vi "Update.vi"(8 "error in (no error)":errorcluster, 11 "Example Source in":refnum<class "Example Source.lvclass">) -> (0 "error out":errorcluster, 3 "Example Source out":refnum<class "Example Source.lvclass">)   [LabVIEW 2020, in "Example Source.lvlib" / "Example Source.lvclass"]
uses:
  Example Source.lvclass
  C:/Program Files/National Instruments/LabVIEW 2020/vi.lib/ActorFramework/Actor/Actor.lvclass
  Timestamp/Timestamp.lvclass
  C:/Users/huipeng8/Desktop/Event-Source-Actor/Source/Template Source/Event Data/Event Data.lvclass
  Doublo Array/Doublo Array.lvclass
  <vilib>/ActorFramework/Actor/Actor.lvclass/Actor.ctl
  <vilib>/ActorFramework/Message Enqueuer/Message Enqueuer.lvclass/Message Enqueuer.ctl
  Timestamp/Timestamp.lvclass/Timestamp.ctl
  Doublo Array/Doublo Array.lvclass/Doublo Array.ctl
  Source/Template Source/Event Source Messages/Generate Event Msg/Generate Event Msg.lvclass/Generate Event Msg.ctl
  <vilib>/ActorFramework/Message Enqueuer/Init from Existing Queue.vi
  <vilib>/ActorFramework/Message Enqueuer/Enqueue.vi
  Source/Template Source/Event Source Messages/Generate Event Msg/Generate Event Msg.lvclass
  C:/Program Files/National Instruments/LabVIEW 2020/vi.lib/ActorFramework/Message/Message.lvclass
  <vilib>/ActorFramework/Message Priority Queue/Priority Enqueue.vi
  <vilib>/ActorFramework/Message Enqueuer/Message Enqueuer.lvclass
  <vilib>/ActorFramework/Actor/Actor.lvclass
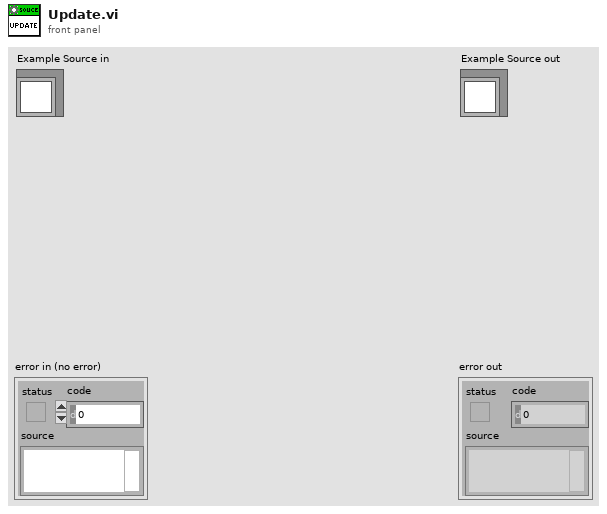
[diagram p1: front panel]
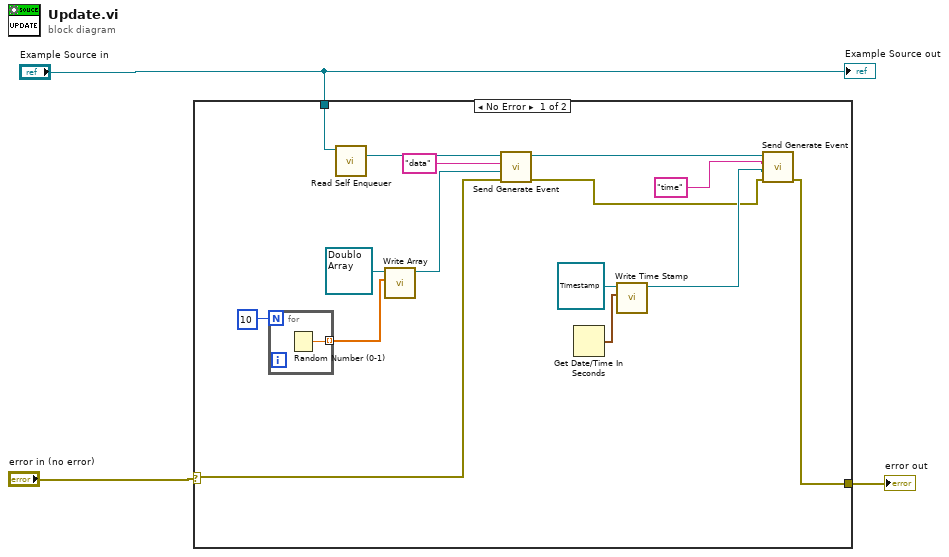
[diagram p0: block diagram]
diagram:
  n1 = case shown="No Error" "error in (no error)" {
    selector: "error in (no error)" -> [w4 w20]
    tunnel: "Example Source in" -> [w13 _]
    tunnel: [w5 w20] -> w2
    frame No Error {
      n2 = for {
        N: 10 -> [_]
        tunnel: [w19] -> w17 mode=indexing
        n3 = Random Number (0-1)() -> (number: 0 to 1=w19:dbl)
      }
      n4 = call <vilib>:"Read Self Enqueuer.vi"("Actor"=w13) -> ("Self Enqueuer"=w12:refnum<class "Message Enqueuer.lvclass">)  [unwired: 10 in]
      n5 = call "Write Array.vi"("Array"=w17, "Doublo Array in"=refnum<class "Doublo Array.lvclass"> refnum ("Example Source.lvlib:Doublo Array.lvclass")) -> ("Doublo Array out"=w10:refnum<class "Doublo Array.lvclass">)  [unwired: 8 in, 1 out]
      n6 = call "Send Generate Event.vi"("error in"=w4, "Event Data"=w10, "Event Name"="data", "Message Enqueuer"=w12) -> ("error out"=w6:errorcluster, "Message Enqueuer out"=w9:refnum<class "Message Enqueuer.lvclass">)  [unwired: 6 in]
      n7 = Get Date/Time In Seconds() -> (seconds since 1Jan1904=w14:timestamp)
      n8 = call "Write Time Stamp.vi"("Time Stamp"=w14, "time in"=refnum<class "Timestamp.lvclass"> refnum ("Example Source.lvlib:time.lvclass")) -> ("time out"=w7:refnum<class "Timestamp.lvclass">)  [unwired: 8 in, 1 out]
      n9 = call "Send Generate Event.vi"("error in"=w6, "Event Data"=w7, "Event Name"="time", "Message Enqueuer"=w9) -> ("error out"=w5:errorcluster)  [unwired: 6 in, 1 out]
    }
    frame Error {
    }
  }
  "error out" <- w2
  "Example Source out" <- "Example Source in"
